vi "Panel at Index.vi"(7 "Type (ArrayPanel)":refnum<class "ArrayPanel.lvclass">, 8 "error in (no error)":errorcluster, 10 "Index":i32, 11 "PanelArray in":refnum<class "ArrayManager.lvclass">) -> (0 "error out":errorcluster, 2 "Panel":refnum<class "ArrayPanel.lvclass">, 3 "PanelArray out":refnum<class "ArrayManager.lvclass">)   [LabVIEW 2020, in "OOPanel.lvlib" / "ArrayManager.lvclass"]
uses:
  ArrayManager.lvclass
  ArrayPanel/ArrayPanel.lvclass
  ArrayManager.lvclass/ArrayManager.ctl
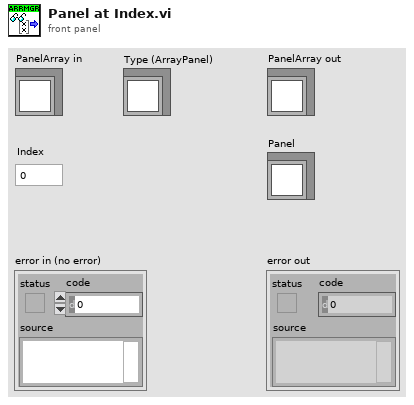
[diagram p1: front panel]
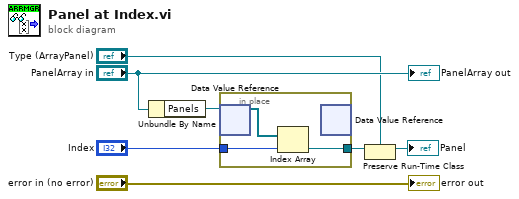
[diagram p0: block diagram]
diagram:
  n1 = Unbundle By Name("PanelArray in") -> ("Panels"=w6:refnum<data-value>)
  n2 = in-place {
    in-place-border: "Index" -> [w9]
    in-place-border: [w8] -> w3
    n3 = in-place-dvr #1(w6) -> (w10:refnum<class "ArrayPanel.lvclass">[])  [unwired: 1 out]
    n4 = Index Array(array=w10, index=w9) -> (element=w8:refnum<class "ArrayPanel.lvclass">)
    n5 = in-place-dvr #1() -> ()  [unwired: 1 in, 2 out]
  }
  n6 = Preserve Run-Time Class(object in=w3, 2:"Type (ArrayPanel)") -> (object out=→"Panel":refnum<class "ArrayPanel.lvclass">)  [unwired: 1 in, 1 out]
  "error out" <- "error in (no error)"
  "PanelArray out" <- "PanelArray in"
